vi "Tools_String Write Entire File.vi"(5 "convert eoln (F)":bool, 8 "error in (no error)":errorcluster, 10 "data":string, 11 "path":path) -> (0 "error out":errorcluster, 3 "duplicate path":path)   [LabVIEW 2017]
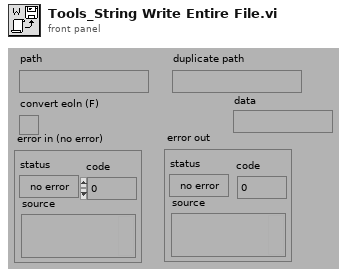
[diagram p1: front panel]
types:
  T1 = enum16{"open", "replace", "create", "open or create", "replace or create", "replace or create with confirmation"}
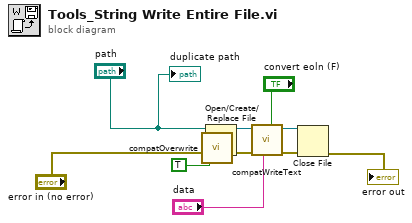
[diagram p0: block diagram]
diagram:
  n1 = call <vilib>:"compatOverwrite.vi"("overwrite (F)"=TRUE) -> ("overwrite?"=w1:T1)
  n2 = Open/Create/Replace File(file path (use dialog)="path", error in="error in (no error)", operation (0:open)=w1) -> (refnum out=w6:refnum<file>, error out=w5:errorcluster)  [unwired: 4 out]
  n3 = call <vilib>:"compatWriteText.vi"("convert eol (F)"="convert eoln (F)", "data"="data", "error in"=w5, "refnum"=w6) -> ("error out"=w10:errorcluster, "dup refnum"=w11:refnum<file>)  [unwired: 1 in, 5 out]
  n4 = Close File(refnum=w11, error in=w10) -> (error out=→"error out":errorcluster)  [unwired: 1 out]
  "duplicate path" <- "path"
